vi "UART2 Write.vi"(8 "Error In":errorcluster, 10 "Data":string, 11 "ChipKit Resource 2":T1={"COM Port"="", "Board Type"=enum."ChipKit uC32", "Connection Type"=enum."USB / Serial", "Baud Rate (115200)"=15, "Bytes Per Packet (15)"=15}) -> (0 "Error Out":errorcluster, 3 "ChipKit Resource":T1={"COM Port"="", "Board Type"=enum."ChipKit uC32", "Connection Type"=enum."USB / Serial", "Baud Rate (115200)"=15, "Bytes Per Packet (15)"=15})   [LabVIEW 2011, in "LabVIEW Interface for ChipKit.lvlib"]
uses:
  LabVIEW Interface for ChipKit.lvlib
  Private/Type Defs/Chipkit Resource.ctl
  Private/Type Defs/Board Type.ctl
  Private/Type Defs/Connection Type.ctl
  Private/Type Defs/Command.ctl
panel:
  out "Read Buffer":string
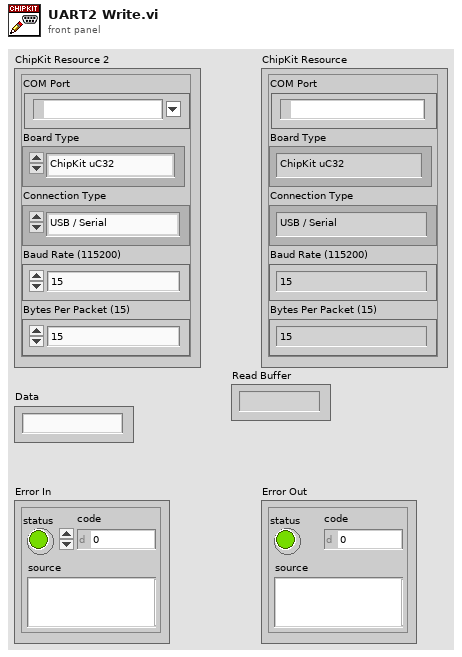
[diagram p1: front panel]
types:
  T1 = typedef "LabVIEW Interface for ChipKit.lvlib/Chipkit Resource.ctl" = cluster{"COM Port":refnum<visa-resource-name>, "Board Type":T2, "Connection Type":T3, "Baud Rate (115200)":u32, "Bytes Per Packet (15)":u32}
  T2 = typedef "LabVIEW Interface for ChipKit.lvlib/Board Type.ctl" = enum16{"ChipKit uC32", "ChipKit Uno32", "ChipKit Max32"}
  T3 = typedef "LabVIEW Interface for ChipKit.lvlib/Connection Type.ctl" = enum8{"USB / Serial", "XBEE", "BlueSmirf (Bluetooth)"}
  T4 = typedef "LabVIEW Interface for ChipKit.lvlib/Command.ctl" = enum8{"setArduinoMode", "flushSerial", "setPinMode", "digitalWritePin", "digitalWritePort", "tone", "digitalReadPin", "digitalReadPort", "analogReadPin", "analogReadPort", "pwmWritePin", "pwmWritePort", "sevenSegment_Configure", "sevenSegment_Write", "I2C Init", "I2C Write", "I2C Read", "SPI Init", "SPI Set Bit Order", "SPI Set Clock Divider", "SPI Set Data Mode", "SPI Send / Receive", "SPI Close", "Servo Set Num Servos", "Servo Config Servo", "Servo Write Angle", "Servo Read Angle", "Servo Write Pulse Width", "Servo Read Pulse Width", "Servo Detach", "LCD Init", "LCD Set Size", "LCD Set Cursor Mode", "LCD Clear", "LCD Set Cursor Position", "LCD Print", "LCD Display Power", "LCD Scroll Display", "LCD Autoscroll", "LCD Print Direction", "LCD Create Custom Char", "LCD Print Custom Char", "contAcqOn", "contAcqOff", "getFirmwareVersion", "FiniteSampleStart", "NA", "NA2", "Conifg Stepper", "Stepper Write", "Stepper Detach", "Stepper Steps To Go", "Config DO Port", "Config DI Port", "UART2 Open", "UART2 Write", "UART2 Bytes Available", "UART2 Read"}
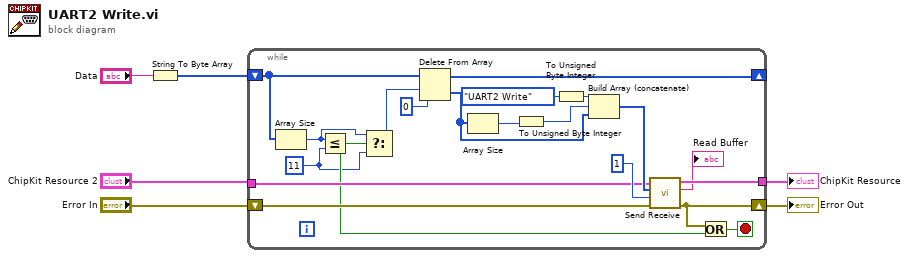
[diagram p0: block diagram]
diagram:
  n1 = String To Byte Array(string="Data") -> (unsigned byte array=w5:u8[])
  n2 = while {
    shift-right: [w22] -> w1
    shift-left: "Error In" -> [w23]
    tunnel: "ChipKit Resource 2" -> [w21]
    tunnel: [w20] -> w2
    shift-right: [w18] -> _
    shift-left: w5 -> [w16]
    stop <- w24 stop-if-true
    w13 = 11 ("length")
    n3 = Array Size(array=w16) -> (size(s)=w14:i32)
    n4 = Less Or Equal?(x=w14, y=w13) -> (x <= y?=w15:bool)
    n5 = Select(t=w14, s=w15, f=w13) -> (s? t:f=w12:i32)
    n6 = Delete From Array(array=w16, length=w12, index=0) -> (deleted portion=w17:u8[], array with subset deleted=w18:u8[])
    n7 = Array Size(array=w17) -> (size(s)=w11:i32)
    n8 = To Unsigned Byte Integer(number=w11) -> (unsigned 8bit integer=w10:u8)
    n9 = To Unsigned Byte Integer(number=Command."UART2 Write" ("Command")) -> (unsigned 8bit integer=w8:u8)
    n10 = Build Array (concatenate)(w8, w10, w17) -> (w25:u8[])
    n11 = call "Send Receive.vi"("Error In"=w23, "Bytes To Read (0)"=u32 1, "Data"=w25, "ChipKit Resource"=w21) -> ("Error Out"=w22:errorcluster, "Read Buffer"=→"Read Buffer":string, "ChipKit Resource"=w20:T1)  [unwired: 5 in]
    n12 = Or(x=w22, y=w15) -> (x .or. y?=w24:bool)
  }
  "Error Out" <- w1
  "ChipKit Resource" <- w2
